vi "Increment Filename.vi"(1 "Filename In":string) -> (0 "Filename Out":string)   [LabVIEW 2019]
doc: "Searches the filename for (XXXX.23) dot separator and a number following. If found, increments the number. If not, appends a dot and a one.\nScott Hannahs, FBNML, Feb 1992"
uses:
  <vilib>/regexp/Match Regular Expression.xnode
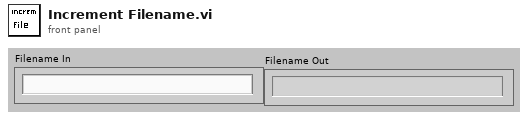
[diagram p1: front panel]
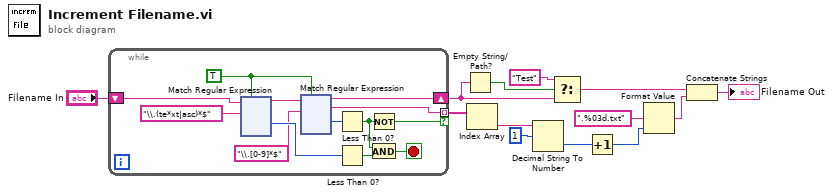
[diagram p0: block diagram]
diagram:
  n1 = while {
    shift-right: [w20] -> w4
    shift-left: "Filename In" -> [w26]
    tunnel: [w16] -> w3 mode=indexing if=w15
    stop <- w17 stop-if-true
    w19 = TRUE ("ignore case? (F)")
    n2 = xnode "Match Regular Expression"("input string"=w26, "regular expression"="\\.(te*xt|asc)*$", "ignore case? (F)"=w19) -> ("before match"=w21:string, "offset past match"=w23:i32)  [unwired: 3 in, 3 out]
    n3 = xnode "Match Regular Expression"("input string"=w21, "regular expression"="\\.[0-9]*$", "ignore case? (F)"=w19) -> ("before match"=w20:string, "whole match"=w16:string, "offset past match"=w18:i32)  [unwired: 3 in, 2 out]
    n4 = Less Than 0?(x=w18) -> (x < 0?=w14:bool)
    n5 = Less Than 0?(x=w23) -> (x < 0?=w24:bool)
    n6 = Not(x=w14) -> (.not. x?=w15:bool)
    n7 = And(x=w14, y=w24) -> (x .and. y?=w17:bool)
  }
  n8 = Empty String/Path?(string/path=w4) -> (empty?=w8:bool)
  n9 = Index Array(array=w3) -> (element=w1:string)  [unwired: 1 in]
  n10 = Decimal String To Number(string=w1, offset=1) -> (number=w9:i32)  [unwired: 1 in, 1 out]
  n11 = Select(t="Test", s=w8, f=w4) -> (s? t:f=w6:string)
  n12 = Increment(x=w9) -> (x+1=w2:i32)
  n13 = Format Value(format string=".%03d.txt", value (0)=w2) -> (output string=w13:string)  [unwired: 1 in]
  n14 = Concatenate Strings(w6, w13) -> (→"Filename Out":string)
